vi "通过棋盘获取可能性索引.vi"(1 "输入的棋盘":T1) -> (0 "索引":i32)   [LabVIEW 2017]
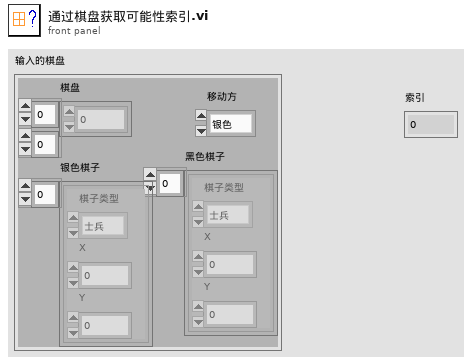
[diagram p1: front panel]
types:
  T1 = cluster{"棋盘":u16[][], "银色棋子":cluster{"棋子类型":enum16{"士兵", "骑士", "主教", "战车", "皇后", "国王", "空"}, "X":u8, "Y":u8}[], "黑色棋子":cluster{"棋子类型":enum16{"士兵", "骑士", "主教", "战车", "皇后", "国王", "空"}, "X":u8, "Y":u8}[], "移动方":enum16{"银色", "黑色"}}
  T2 = cluster{"棋盘":u16[][], "银色棋子":cluster{"棋子类型":enum16{"士兵", "骑士", "主教", "战车", "皇后", "国王", "空"}, "X":u8, "Y":u8}[], "黑色棋子":cluster{"棋子类型":enum16{"士兵", "骑士", "主教", "战车", "皇后", "国王", "空"}, "X":u8, "Y":u8}[], "移动方":enum16{"银色", "黑色"}}[]
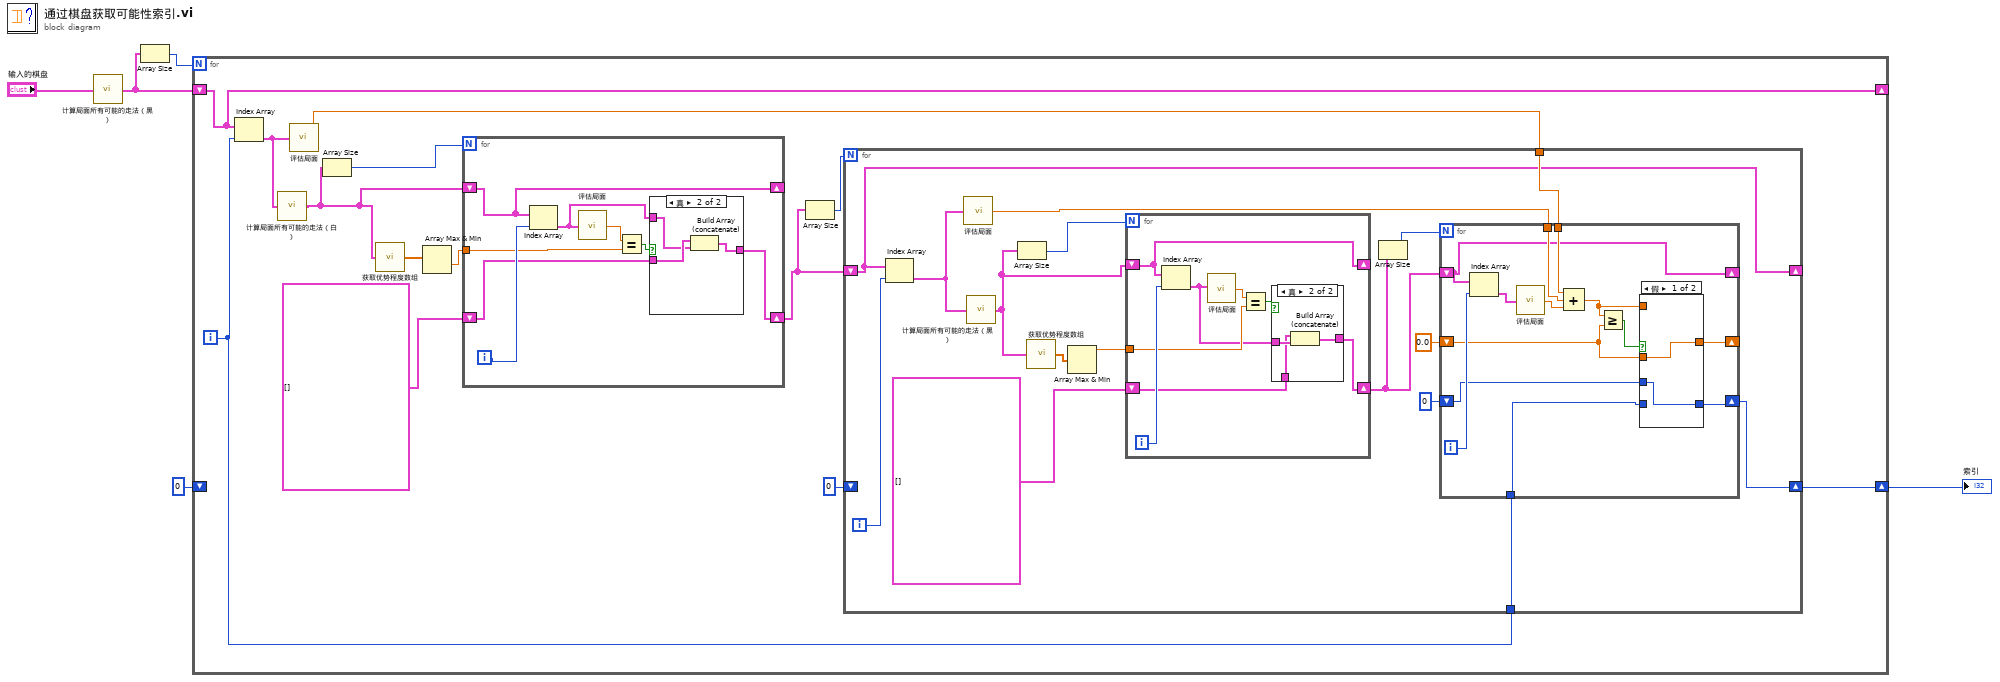
[diagram p0: block diagram]
diagram:
  n1 = call "计算局面所有可能的走法（黑）.vi"("输入的棋盘"="输入的棋盘") -> ("可能移动"=w4:T2)
  n2 = Array Size(array=w4) -> (size(s)=w3:i32)
  n3 = for {
    N: w3 -> [_]
    shift-right: [w18] -> _
    shift-left: w4 -> [w18]
    shift-right: [w6] -> w1
    shift-left: 0 -> [_]
    i -> [w8]
    n4 = Index Array(array=w18, index=w8) -> (element=w17:T1)
    n5 = call "计算局面所有可能的走法（白）.vi"("输入的棋盘"=w17) -> ("可能移动"=w15:T2)
    n6 = call "评估局面.vi"("输入的棋盘"=w17) -> ("优势程度"=w9:dbl)
    n7 = Array Size(array=w15) -> (size(s)=w16:i32)
    n8 = call "获取优势程度数组.vi"("输入数组"=w15) -> ("输出数组"=w14:dbl[])
    n9 = Array Max & Min(array=w14) -> (min value=w13:dbl)  [unwired: 3 out]
    n10 = for {
      N: w16 -> [_]
      shift-right: [w68] -> _
      shift-left: w15 -> [w68]
      tunnel: w13 -> [w69]
      shift-right: [w64] -> w10
      shift-left: T2 [] -> [w65]
      i -> [w71]
      n11 = Index Array(array=w68, index=w71) -> (element=w66:T1)
      n12 = call "评估局面.vi"("输入的棋盘"=w66) -> ("优势程度"=w70:dbl)
      n13 = Equal?(x=w70, y=w69) -> (x = y?=w67:bool)
      n14 = case shown="真" w67 {
        tunnel: w66 -> [_ w74]
        tunnel: w65 -> [w72 w75]
        tunnel: [w72 w73] -> w64
        frame False {
        }
        frame True {
          n15 = Build Array (concatenate)(w75, w74) -> (w73:T2)
        }
      }
    }
    n16 = Array Size(array=w10) -> (size(s)=w11:i32)
    n17 = for {
      N: w11 -> [_]
      shift-right: [w23] -> _
      shift-left: w10 -> [w23]
      tunnel: w9 -> [w25]
      tunnel: w8 -> [w22]
      shift-right: [w19] -> w6
      shift-left: 0 -> [_]
      i -> [w34]
      n18 = Index Array(array=w23, index=w34) -> (element=w33:T1)
      n19 = call "评估局面.vi"("输入的棋盘"=w33) -> ("优势程度"=w24:dbl)
      n20 = call "计算局面所有可能的走法（黑）.vi"("输入的棋盘"=w33) -> ("可能移动"=w29:T2)
      n21 = Array Size(array=w29) -> (size(s)=w32:i32)
      n22 = call "获取优势程度数组.vi"("输入数组"=w29) -> ("输出数组"=w31:dbl[])
      n23 = Array Max & Min(array=w31) -> (max value=w30:dbl)  [unwired: 3 out]
      n24 = for {
        N: w32 -> [_]
        tunnel: w30 -> [w57]
        shift-right: [w56] -> _
        shift-left: w29 -> [w56]
        shift-right: [w53] -> w26
        shift-left: T2 [] -> [w54]
        i -> [w59]
        n25 = Index Array(array=w56, index=w59) -> (element=w55:T1)
        n26 = call "评估局面.vi"("输入的棋盘"=w55) -> ("优势程度"=w58:dbl)
        n27 = Equal?(x=w58, y=w57) -> (x = y?=w52:bool)
        n28 = case shown="真" w52 {
          tunnel: w55 -> [_ w63]
          tunnel: w54 -> [w60 w62]
          tunnel: [w60 w61] -> w53
          frame False {
          }
          frame True {
            n29 = Build Array (concatenate)(w62, w63) -> (w61:T2)
          }
        }
      }
      n30 = Array Size(array=w26) -> (size(s)=w27:i32)
      n31 = for {
        N: w27 -> [_]
        shift-right: [w42] -> _
        shift-left: w26 -> [w42]
        tunnel: w25 -> [w44]
        tunnel: w24 -> [w43]
        shift-right: [w39] -> _
        shift-left: 0.0 -> [w38]
        tunnel: w22 -> [w37]
        shift-right: [w36] -> w19
        shift-left: 0 -> [w35]
        i -> [w47]
        n32 = Index Array(array=w42, index=w47) -> (element=w46:T1)
        n33 = call "评估局面.vi"("输入的棋盘"=w46) -> ("优势程度"=w45:dbl)
        n34 = Compound Arithmetic op=ADD(w44, w43, w45) -> (w40:dbl)
        n35 = Greater Or Equal?(x=w40, y=w38) -> (x >= y?=w41:bool)
        n36 = case shown="假" w41 {
          tunnel: w40 -> [_ w51]
          tunnel: [w49 w51] -> w39
          tunnel: w38 -> [w49 _]
          tunnel: w37 -> [_ w50]
          tunnel: [w48 w50] -> w36
          tunnel: w35 -> [w48 _]
          frame False {
          }
          frame True {
          }
        }
      }
    }
  }
  "索引" <- w1
